vi "monthly_loan.vi"() -> ()   [LabVIEW 2020]
panel:
  out "monthly payment":dbl
  in  "interest rate":dbl
  in  "no. of months":dbl
  in  "loan amount":dbl
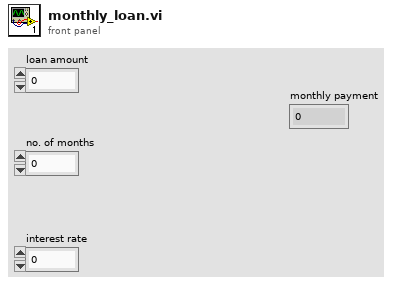
[diagram p1: front panel]
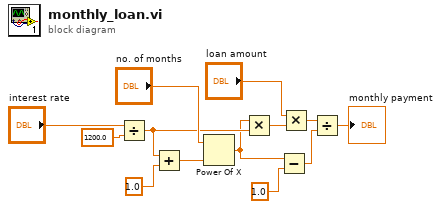
[diagram p0: block diagram]
diagram:
  n1 = Divide(x="interest rate", y=1200.0) -> (x/y=w6:dbl)
  n2 = Add(x=w6, y=1.0) -> (x+y=w4:dbl)
  n3 = Power Of X(1:w4, 2:"no. of months") -> (0:w2:dbl)
  n4 = Multiply(x=w2, y=w6) -> (x*y=w9:dbl)
  n5 = Subtract(x=w2, y=1.0) -> (x-y=w1:dbl)
  n6 = Multiply(x="loan amount", y=w9) -> (x*y=w8:dbl)
  n7 = Divide(x=w8, y=w1) -> (x/y=→"monthly payment":dbl)
